vi "setTiming.vi"(2 "error in (no error)":errorcluster, 3 "niDAQmxAO in":refnum<class "niDAQmxAO.lvclass">) -> (0 "error out":errorcluster, 1 "niDAQmxAO out":refnum<class "niDAQmxAO.lvclass">)   [LabVIEW 2009, in "Hardware.lvlib" / "Channels.lvlib" / "niDAQmxAO.lvclass"]
uses:
  niDAQmxAO.lvclass
  <vilib>/DAQmx/configure/timing.llb/DAQmx Timing (Sample Clock).vi
  <vilib>/DAQmx/configure/trigger.llb/DAQmx Start Trigger (Digital Edge).vi
  niDAQmxAO.lvclass/niDAQmxAO.ctl
  C:/Program Files/National Instruments/LabVIEW 2009/resource/objmgr/daqmx.rc
  AnalogOutput.lvclass
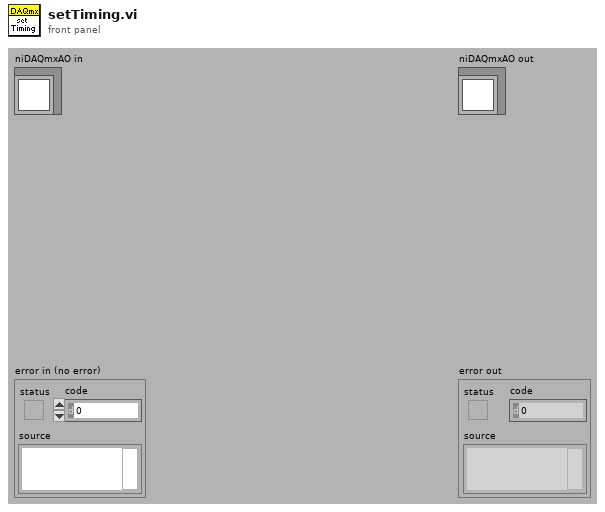
[diagram p1: front panel]
types:
  T1 = cluster{"Clock source":string, "Clock rate":dbl, "Start trigger line":string, "Sample Rate":dbl, "Sample No.":dbl}
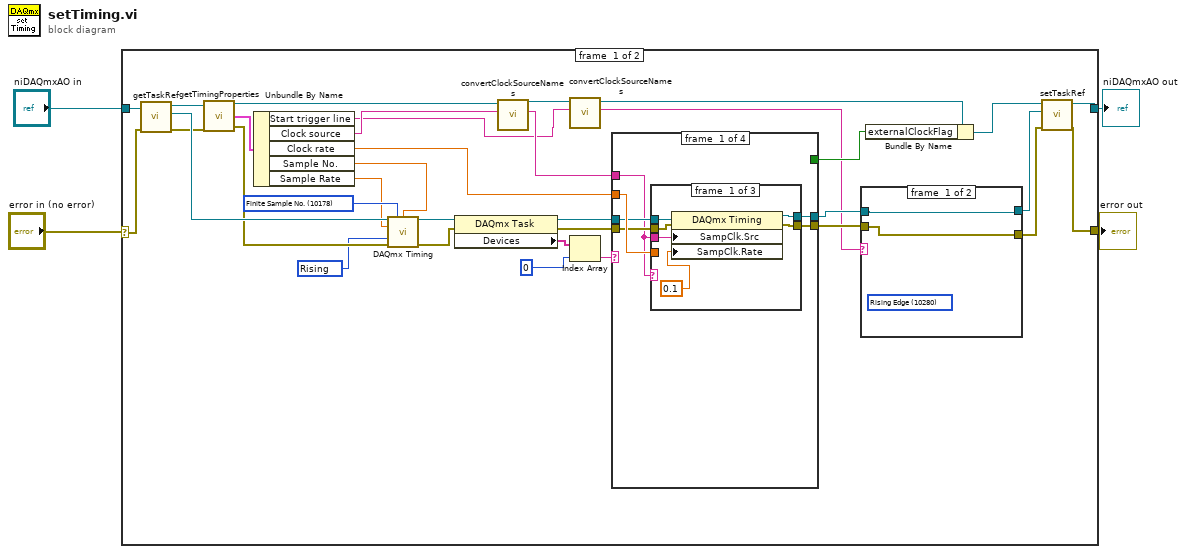
[diagram p0: block diagram]
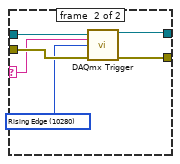
[diagram p2: hidden frame]
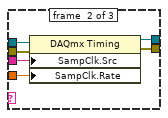
[diagram p3: hidden frame]
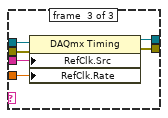
[diagram p4: hidden frame]
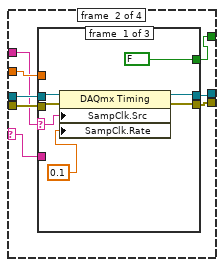
[diagram p5: hidden frame]
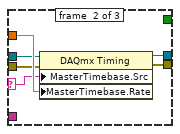
[diagram p6: hidden frame]
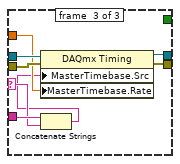
[diagram p7: hidden frame]
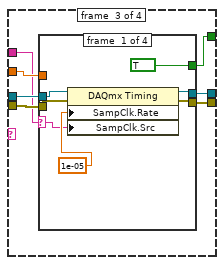
[diagram p8: hidden frame]
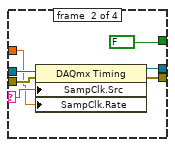
[diagram p9: hidden frame]
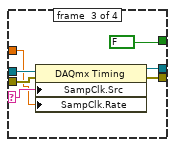
[diagram p10: hidden frame]
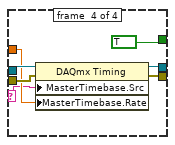
[diagram p11: hidden frame]
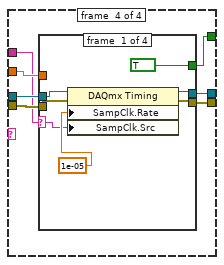
[diagram p12: hidden frame]
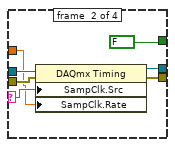
[diagram p13: hidden frame]
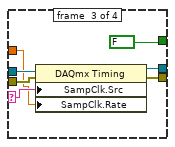
[diagram p14: hidden frame]
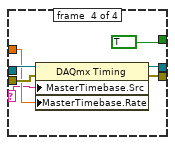
[diagram p15: hidden frame]
diagram:
  n1 = case shown="No Error" "error in (no error)" {
    selector: "error in (no error)" -> [w29 w171]
    tunnel: [w26 w171] -> w3
    tunnel: [w25 w170] -> w1
    tunnel: "niDAQmxAO in" -> [w38 w170]
    frame #0 {
      w13 = u16 10178 items=["Finite Sample No."=10178]
      w15 = 10280 items=["Rising"=10280, "Falling"=10171] ("active edge")
      n2 = call "getTaskRef.vi"("error in (no error)"=w29, "niDAQmxAO.lvclass in"=w38) -> ("error out"=w32:errorcluster, "DAQmx Task Ref"=w37:refnum<k21>, "niDAQmxAO.lvclass out"=w30:refnum<class "niDAQmxAO.lvclass">)  [unwired: 7 in]
      n3 = call "getTimingProperties.vi"("AnalogOutput.lvclass in"=w30, "error in (no error)"=w32) -> ("AnalogOutput.lvclass out"=w17:refnum<class "niDAQmxAO.lvclass">, "Timing"=w34:T1, "error out"=w31:errorcluster)
      n4 = Unbundle By Name(w34) -> ("Start trigger line"=w8:string, "Clock source"=w16:string, "Clock rate"=w33:dbl, "Sample No."=w5:dbl, "Sample Rate"=w10:dbl)
      n5 = call-poly <vilib>:"DAQmx Timing.vi"("task/channels in"=w37, "sample mode"=w13, "samples per channel"=w5, "rate"=w10, "active edge"=w15, "error in"=w31) -> ("task out"=w24:refnum<k21>, "error out"=w23:errorcluster)  [unwired: 8 in]
      n6 = property class="DAQmx Task"(reference=w24, error in=w23) -> (reference out=w20:refnum<k21>, error out=w19:errorcluster, "Devices"=w21:tag[])
      n7 = call "convertClockSourceNames.vi"("Clock Source"=w16, "AnalogOutput in"=w17) -> ("convertedClockName"=w14:string, "AnalogOutput out"=w9:refnum<class "niDAQmxAO.lvclass">)  [unwired: 7 in, 1 out]
      n8 = call "convertClockSourceNames.vi"("Clock Source"=w8, "AnalogOutput in"=w9) -> ("convertedClockName"=w7:string, "AnalogOutput out"=w6:refnum<class "niDAQmxAO.lvclass">)  [unwired: 7 in, 1 out]
      n9 = Index Array(array=w21, index=0) -> (element=w18:tag)
      n10 = case shown="\"UsbDAQ\"" w18 {
        selector: w18 -> [_ w72 _ _]
        tunnel: [w52 w78 w106 w141] -> w36
        tunnel: [w51 w77 w105 w140] -> w35
        tunnel: w33 -> [w50 w76 w102 w137]
        tunnel: w14 -> [w47 w73 w101 w136]
        tunnel: w20 -> [w49 w75 w104 w139]
        tunnel: w19 -> [w48 w74 w103 w138]
        tunnel: [_ w71 w100 w135] -> w11
        frame #0 {
          n11 = case shown="\"OnboardClock\", \"internal\", \"none\"" w47 {
            tunnel: [w57 w64 w70] -> w52
            tunnel: [w56 w63 w69] -> w51
            tunnel: w50 -> [_ w62 w68]
            tunnel: w47 -> [w55 w61 w67]
            tunnel: w49 -> [w58 w60 w66]
            tunnel: w48 -> [w54 w59 w65]
            frame #0 {
              n12 = property class="DAQmx Timing"(reference=w58, error in=w54, "SampClk.Src"=w55, "SampClk.Rate"=0.1) -> (reference out=w57:refnum<k21>, error out=w56:errorcluster)
            }
            frame #1 {
              n13 = property class="DAQmx Timing"(reference=w60, error in=w59, "SampClk.Src"=w61, "SampClk.Rate"=w62) -> (reference out=w64:refnum<k21>, error out=w63:errorcluster)
            }
            frame #2 {
              n14 = property class="DAQmx Timing"(reference=w66, error in=w65, "RefClk.Src"=w67, "RefClk.Rate"=w68) -> (reference out=w70:refnum<k21>, error out=w69:errorcluster)
            }
          }
        }
        frame #1 {
          n15 = case shown="\"OnboardClock\", \"internal\", \"none\"" w73 {
            selector: w73 -> [w81 w86 w93]
            tunnel: [w83 w91 w97] -> w78
            tunnel: [w82 w90 w96] -> w77
            tunnel: w76 -> [_ w89 w95]
            tunnel: w75 -> [w85 w88 w99]
            tunnel: w74 -> [w84 w87 w98]
            tunnel: w72 -> [_ _ w94]
            tunnel: [FALSE _ _] -> w71
            frame #0 {
              n16 = property class="DAQmx Timing"(reference=w85, error in=w84, "SampClk.Src"=w81, "SampClk.Rate"=0.1) -> (reference out=w83:refnum<k21>, error out=w82:errorcluster)
            }
            frame #1 {
              n17 = property class="DAQmx Timing"(reference=w88, error in=w87, "MasterTimebase.Src"=w86, "MasterTimebase.Rate"=w89) -> (reference out=w91:refnum<k21>, error out=w90:errorcluster)
            }
            frame #2 {
              n18 = Concatenate Strings(w94, w93) -> (w92:string)
              n19 = property class="DAQmx Timing"(reference=w99, error in=w98, "MasterTimebase.Src"=w92, "MasterTimebase.Rate"=w95) -> (reference out=w97:refnum<k21>, error out=w96:errorcluster)
            }
          }
        }
        frame #2 {
          n20 = case shown="Default" w101 {
            selector: w101 -> [w108 w118 w125 w129]
            tunnel: [w113 w120 w127 w134] -> w106
            tunnel: [w112 w119 w126 w133] -> w105
            tunnel: w104 -> [w111 w117 w124 w132]
            tunnel: w103 -> [w110 w116 w123 w131]
            tunnel: w102 -> [_ w115 w121 w130]
            tunnel: [TRUE FALSE FALSE TRUE] -> w100
            frame #0 {
              n21 = property class="DAQmx Timing"(reference=w111, error in=w110, "SampClk.Rate"=1e-05, "SampClk.Src"=w108) -> (reference out=w113:refnum<k21>, error out=w112:errorcluster)
            }
            frame #1 {
              n22 = property class="DAQmx Timing"(reference=w117, error in=w116, "SampClk.Src"=w118, "SampClk.Rate"=w115) -> (reference out=w120:refnum<k21>, error out=w119:errorcluster)
            }
            frame #2 {
              n23 = property class="DAQmx Timing"(reference=w124, error in=w123, "SampClk.Src"=w125, "SampClk.Rate"=w121) -> (reference out=w127:refnum<k21>, error out=w126:errorcluster)
            }
            frame #3 {
              n24 = property class="DAQmx Timing"(reference=w132, error in=w131, "MasterTimebase.Src"=w129, "MasterTimebase.Rate"=w130) -> (reference out=w134:refnum<k21>, error out=w133:errorcluster)
            }
          }
        }
        frame #3 {
          n25 = case shown="\"internal\"" w136 {
            selector: w136 -> [w143 w153 w160 w164]
            tunnel: [w148 w155 w162 w169] -> w141
            tunnel: [w147 w154 w161 w168] -> w140
            tunnel: w139 -> [w146 w152 w159 w167]
            tunnel: w138 -> [w145 w151 w158 w166]
            tunnel: w137 -> [_ w150 w156 w165]
            tunnel: [TRUE FALSE FALSE TRUE] -> w135
            frame #0 {
              n26 = property class="DAQmx Timing"(reference=w146, error in=w145, "SampClk.Rate"=1e-05, "SampClk.Src"=w143) -> (reference out=w148:refnum<k21>, error out=w147:errorcluster)
            }
            frame #1 {
              n27 = property class="DAQmx Timing"(reference=w152, error in=w151, "SampClk.Src"=w153, "SampClk.Rate"=w150) -> (reference out=w155:refnum<k21>, error out=w154:errorcluster)
            }
            frame #2 {
              n28 = property class="DAQmx Timing"(reference=w159, error in=w158, "SampClk.Src"=w160, "SampClk.Rate"=w156) -> (reference out=w162:refnum<k21>, error out=w161:errorcluster)
            }
            frame #3 {
              n29 = property class="DAQmx Timing"(reference=w167, error in=w166, "MasterTimebase.Src"=w164, "MasterTimebase.Rate"=w165) -> (reference out=w169:refnum<k21>, error out=w168:errorcluster)
            }
          }
        }
      }
      n30 = case shown="Default" w7 {
        selector: w7 -> [_ w41]
        tunnel: w36 -> [w40 w46]
        tunnel: w35 -> [w39 w45]
        tunnel: [w40 w43] -> w28
        tunnel: [w39 w42] -> w27
        frame #0 {
          (unwired) u16 10280 items=["Rising Edge"=10280]
        }
        frame #1 {
          w44 = u16 10280 items=["Rising Edge"=10280]
          n31 = call-poly <vilib>:"DAQmx Trigger.vi"("task/channels in"=w46, "source"=w41, "edge"=w44, "error in"=w45) -> ("task out"=w43:refnum<k21>, "error out"=w42:errorcluster)  [unwired: 10 in]
        }
      }
      n32 = Bundle By Name(cluster=w6, "externalClockFlag"=w11) -> (w12:refnum<class "niDAQmxAO.lvclass">)
      n33 = call "setTaskRef.vi"("error in (no error)"=w27, "DAQmx Task Ref"=w28, "niDAQmxAO.lvclass in"=w12) -> ("error out"=w26:errorcluster, "niDAQmxAO.lvclass out"=w25:refnum<class "niDAQmxAO.lvclass">)  [unwired: 7 in]
    }
    frame #1 {
    }
  }
  "error out" <- w3
  "niDAQmxAO out" <- w1
